vi "clqr.vi"(8 "R":T1=[[1.0]], 9 "Q":T1=[[100.0, 0.0], [0.0, 10.0]], 10 "B":T1=[[0.0], [1.0]], 11 "A":T1=[[0.0, 1.0], [0.0, -1.0]]) -> (3 "K":T1=[[-1.0000000000000027, -1.0000000000000129]])   [LabVIEW 2017]
uses:
  <vilib>/Analysis/Matrix/Datatypes/RealMatrix.ctl
  <vilib>/Analysis/baseanly.llb/Complex A x B.vi
  <vilib>/Analysis/baseanly.llb/Real Inverse Matrix.vi
  <vilib>/Analysis/NI_AALBase.lvlib
  <vilib>/Analysis/Matrix/NI_Matrix.lvlib
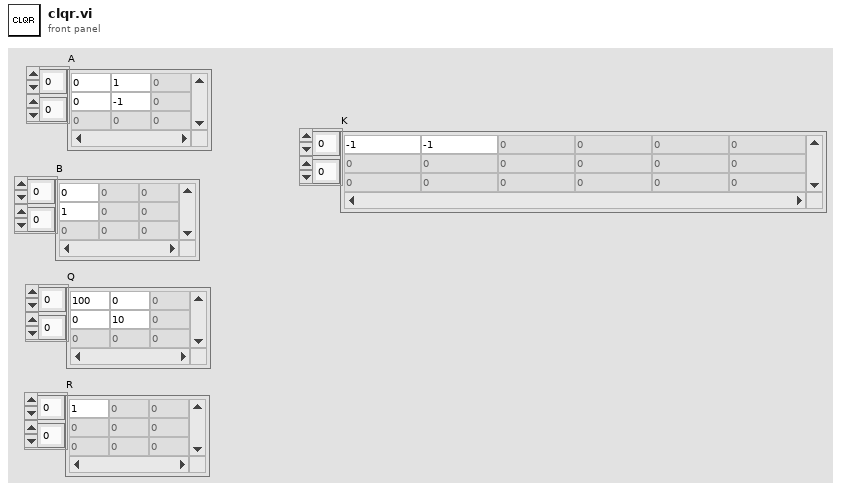
[diagram p1: front panel]
types:
  T1 = typedef "NI_Matrix.lvlib/RealMatrix.ctl" = dbl[][]
  T2 = typedef "NI_Matrix.lvlib/ComplexMatrix.ctl" = cdb[][]
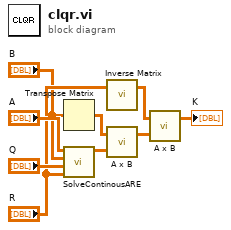
[diagram p0: block diagram]
diagram:
  n1 = Transpose Matrix(1:"B") -> (0:w5:T1)
  n2 = call "SolveContinousARE.vi"("R"="R", "Q"="Q", "B"="B", "A"="A") -> ("A x B"=w4:T2)  [unwired: 7 in]
  n3 = call-poly <vilib>:"Inverse Matrix.vi"("Input Matrix"="R") -> ("Inverse Matrix"=w3:T1)  [unwired: 1 in, 1 out]
  n4 = call-poly <vilib>:"A x B.vi"("B"=w4, "A"=w5) -> ("A x B"=w2:T2)  [unwired: 1 out]
  n5 = call-poly <vilib>:"A x B.vi"("B"=w2, "A"=w3) -> ("A x B"=→"K":T2)  [unwired: 1 out]
